vi "Math-Uniform Loess.vi"(9 "Quadratic?":bool, 10 "Span":i32, 11 "Array":dbl[](array[numeric])) -> (3 "Smoothed Array":dbl[](array[numeric]))   [LabVIEW 2020]
uses:
  LinSpace (x0-dx-npts).vi
  <vilib>/Analysis/7linalg.llb/Real QR Decomposition.vi
  <vilib>/Analysis/7linalg.llb/Real Transpose Matrix.vi
  <vilib>/Analysis/baseanly.llb/Real A x B.vi
  <vilib>/Analysis/2dsp.llb/1D Convolution (DBL).vi
  <vilib>/Analysis/Matrix/Numeric/Conversions/Matrix To Array - RM.vi
  <vilib>/Analysis/NI_AALPro.lvlib
  <vilib>/Analysis/NI_AALBase.lvlib
  <vilib>/Analysis/Matrix/NI_Matrix.lvlib
  <vilib>/Analysis/NI_AALBLAS.lvlib
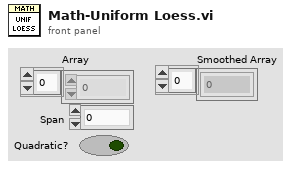
[diagram p1: front panel]
types:
  T1 = typedef "NI_Matrix.lvlib/RealMatrix.ctl" = dbl[][]
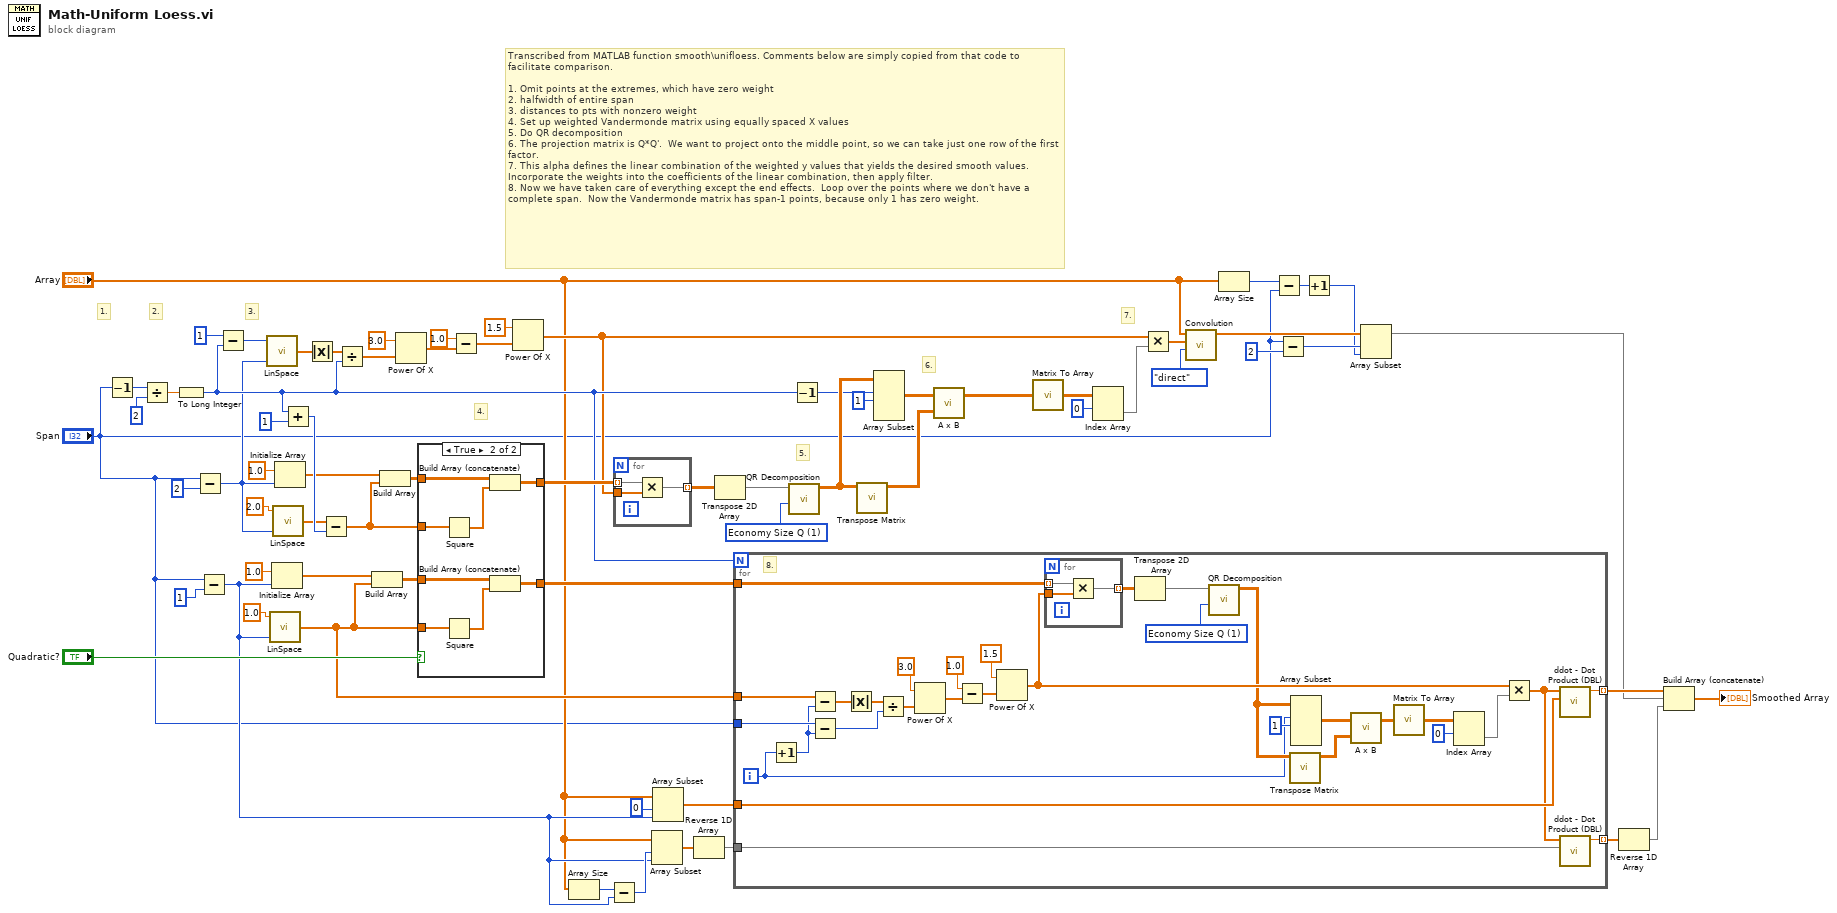
[diagram p0: block diagram]
diagram:
  w47 = u16 1 items=["Full Size Q", "Economy Size Q", "No Q"] ("Q option")
  # "7."
  # "6."
  # "5."
  # "4."
  # "2."
  # "3."
  # "1."
  # "Transcribed from MATLAB function smooth\\unifloess. Comments below are simply copied from that code to facilitate comparison.\n\n1. Omit points at the extremes, which have zero weight\n2. halfwidth of entire span \n3. distances to pts with nonzero weight\n4. Set up weighted Vandermonde matrix using equally spaced X values\n5. Do QR decomposition\n6. The projection matrix is Q*Q'.  We want to project onto the middle point, so we can take just one row of the first factor.\n7. This alpha defines the linear combination of the weighted y values that yields the desired smooth values.  Incorporate the weights into the coefficients of the linear combination, then apply filter.\n8. Now we have taken care of everything except the end effects.  Loop over the points where we don't have a complete span.  Now the Vandermonde matrix has span-1 points, because only 1 has zero weight."
  n1 = Decrement(x="Span") -> (x-1=w67:i32)
  n2 = Divide(x=w67, y=2) -> (x/y=w66:dbl)
  n3 = To Long Integer(number=w66) -> (32bit integer=w26:i32)
  n4 = Subtract(x="Span", y=2) -> (x-y=w8:i32)
  n5 = Subtract(x="Span", y=1) -> (x-y=w15:i32)
  n6 = Subtract(x=1, y=w26) -> (x-y=w64:i32)
  n7 = call-poly "LinSpace.vi"("npts"=w8, "x0"=w64) -> ("Array"=w63:dbl[])  [unwired: 2 in, 1 out]
  n8 = call-poly "LinSpace.vi"("npts"=w15, "x0"=1.0) -> ("Array"=w24:dbl[])  [unwired: 2 in, 1 out]
  n9 = Initialize Array(1.0 ("element"), w15) -> (w25:dbl[])
  n10 = call-poly "LinSpace.vi"("npts"=w8, "x0"=2.0) -> ("Array"=w28:dbl[])  [unwired: 2 in, 1 out]
  n11 = Initialize Array(1.0 ("element"), w8) -> (w29:dbl[])
  n12 = Add(x=w26, y=1) -> (x+y=w30:i32)
  n13 = Absolute Value(x=w63) -> (abs(x)=w59:dbl[])
  n14 = Subtract(x=w28, y=w30) -> (x-y=w27:dbl[])
  n15 = Divide(x=w59, y=w26) -> (x/y=w58:dbl[])
  n16 = Build Array(w25, w24) -> (w32:dbl[][])
  n17 = Build Array(w29, w27) -> (w51:dbl[][])
  n18 = Power Of X(1:w58, 2:3.0) -> (0:w56:dbl[])
  n19 = case shown="True" "Quadratic?" {
    tunnel: w27 -> [_ w77]
    tunnel: w51 -> [w70 w78]
    tunnel: [w70 w75] -> w50
    tunnel: w32 -> [w69 w72]
    tunnel: w24 -> [_ w73]
    tunnel: [w69 w71] -> w23
    frame False {
    }
    frame True {
      n20 = Square(x=w77) -> (x^2=w76:dbl[])
      n21 = Square(x=w73) -> (x^2=w74:dbl[])
      n22 = Build Array (concatenate)(w78, w76) -> (w75:dbl[][])
      n23 = Build Array (concatenate)(w72, w74) -> (w71:dbl[][])
    }
  }
  n24 = Subtract(x=1.0, y=w56) -> (x-y=w55:dbl[])
  n25 = Power Of X(1:w55, 2:1.5) -> (0:w20:dbl[])
  n26 = Array Size(array="Array") -> (size(s)=w17:i32)
  n27 = Subtract(x=w17, y=w15) -> (x-y=w16:i32)
  n28 = for {
    tunnel: w50 -> [w81] mode=indexing
    tunnel: w20 -> [w80]
    tunnel: [w79] -> w49 mode=indexing
    n29 = Multiply(x=w81, y=w80) -> (x*y=w79:dbl[])
  }
  n30 = Array Subset(array="Array", index=w16, length=w15) -> (w19:dbl[])
  n31 = Array Subset(array="Array", index=0, length=w15) -> (w21:dbl[])
  n32 = Reverse 1D Array(array=w19) -> (reversed array=w18:dbl[])
  n33 = Transpose 2D Array(2D array=w49) -> (transposed array=w48:dbl[][])
  n34 = for {
    N: w26 -> [_]
    tunnel: w24 -> [w112]
    tunnel: "Span" -> [w110]
    tunnel: w23 -> [w100]
    tunnel: w21 -> [w86]
    tunnel: w18 -> [w83]
    tunnel: [w85] -> w14 mode=indexing
    tunnel: [w82] -> w13 mode=indexing
    i -> [w87]
    w98 = u16 1 items=["Full Size Q", "Economy Size Q", "No Q"] ("Q option")
    # "8."
    n35 = Increment(x=w87) -> (x+1=w109:i32)
    n36 = Subtract(x=w112, y=w109) -> (x-y=w111:dbl[])
    n37 = Subtract(x=w110, y=w109) -> (x-y=w102:i32)
    n38 = Absolute Value(x=w111) -> (abs(x)=w103:dbl[])
    n39 = Divide(x=w103, y=w102) -> (x/y=w101:dbl[])
    n40 = Power Of X(1:w101, 2:3.0) -> (0:w106:dbl[])
    n41 = Subtract(x=1.0, y=w106) -> (x-y=w105:dbl[])
    n42 = Power Of X(1:w105, 2:1.5) -> (0:w89:dbl[])
    n43 = for {
      tunnel: w100 -> [w115] mode=indexing
      tunnel: w89 -> [w114]
      tunnel: [w113] -> w97 mode=indexing
      n44 = Multiply(x=w115, y=w114) -> (x*y=w113:dbl[])
    }
    n45 = Transpose 2D Array(2D array=w97) -> (transposed array=w99:dbl[][])
    n46 = call-poly <vilib>:"QR Decomposition.vi"("Q option"=w98, "A"=w99) -> ("Q"=w88:T1)  [unwired: 6 in, 3 out]
    n47 = call-poly <vilib>:"Transpose Matrix.vi"("Input Matrix"=w88) -> ("Matrix Transpose"=w96:T1)  [unwired: 9 in, 1 out]
    n48 = Array Subset(array=w88, index (row)=w87, length (row)=1 ("length")) -> (w93:T1)  [unwired: 2 in]
    n49 = call-poly <vilib>:"A x B.vi"("B"=w96, "A"=w93) -> ("A x B"=w95:T1)  [unwired: 1 out]
    n50 = call-poly <vilib>:"Matrix To Array.vi"("Real Matrix"=w95) -> ("Real 2D Array"=w91:dbl[][])
    n51 = Index Array(array=w91, index (row)=0 ("index")) -> (element=w90:dbl[])  [unwired: 1 in]
    n52 = Multiply(x=w89, y=w90) -> (x*y=w84:dbl[])
    n53 = call <vilib>:"ddot - Dot Product (DBL).vi"("y"=w86, "x"=w84) -> ("ddot"=w85:dbl)  [unwired: 8 in, 1 out]
    n54 = call <vilib>:"ddot - Dot Product (DBL).vi"("y"=w83, "x"=w84) -> ("ddot"=w82:dbl)  [unwired: 8 in, 1 out]
  }
  n55 = call-poly <vilib>:"QR Decomposition.vi"("Q option"=w47, "A"=w48) -> ("Q"=w46:T1)  [unwired: 6 in, 3 out]
  n56 = Decrement(x=w26) -> (x-1=w41:i32)
  n57 = call-poly <vilib>:"Transpose Matrix.vi"("Input Matrix"=w46) -> ("Matrix Transpose"=w45:T1)  [unwired: 9 in, 1 out]
  n58 = Array Subset(array=w46, index (row)=w41, length (row)=1 ("length")) -> (w42:T1)  [unwired: 2 in]
  n59 = call-poly <vilib>:"A x B.vi"("B"=w45, "A"=w42) -> ("A x B"=w44:T1)  [unwired: 1 out]
  n60 = call-poly <vilib>:"Matrix To Array.vi"("Real Matrix"=w44) -> ("Real 2D Array"=w39:dbl[][])
  n61 = Index Array(array=w39, index (row)=0 ("index")) -> (element=w38:dbl[])  [unwired: 1 in]
  n62 = Multiply(x=w20, y=w38) -> (x*y=w36:dbl[])
  n63 = call-poly <vilib>:"Convolution.vi"("algorithm"=enum32{"direct", "frequency domain"}."direct", "Y"=w36, "X"="Array") -> ("X * Y"=w12:dbl[])  [unwired: 7 in, 1 out]
  n64 = Array Size(array="Array") -> (size(s)=w6:i32)
  n65 = Subtract(x=w6, y="Span") -> (x-y=w2:i32)
  n66 = Subtract(x="Span", y=2) -> (x-y=w5:i32)
  n67 = Increment(x=w2) -> (x+1=w1:i32)
  n68 = Array Subset(array=w12, index=w5, length=w1) -> (w9:dbl[])
  n69 = Reverse 1D Array(array=w13) -> (reversed array=w11:dbl[])
  n70 = Build Array (concatenate)(w14, w9, w11) -> (→"Smoothed Array":dbl[])
